vi "FTW-Request-ReplyToPoisonPill.vi"(0 "Poison Pill Request":refnum<data-value>, 5 "Shutting Down?":bool=TRUE, 11 "error in":errorcluster) -> (4 "Poison Pill Response":refnum<data-value>, 15 "error out":errorcluster)   [LabVIEW 2014]
doc: "Sends a response message back to the requesting client. This message is attempts to send unconditionally of incoming error. Take caution to wire a sanitized error into this function, because it will be repeated back onto the client. Said another way, an error generated while processing the request will be not only thrown on the request handler, but also on the client as well."
uses:
  json/core/FTW-JSON-Core-Structure.ctl
panel:
  # "Inputs"
  # "Outputs"
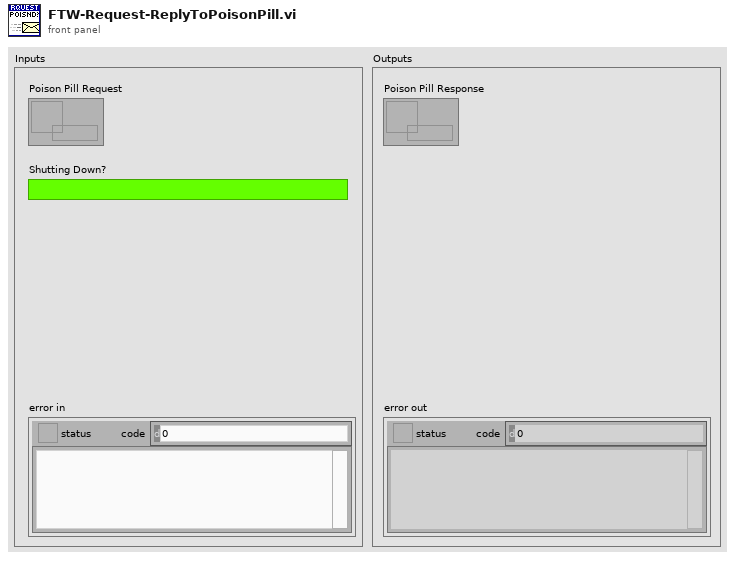
[diagram p1: front panel]
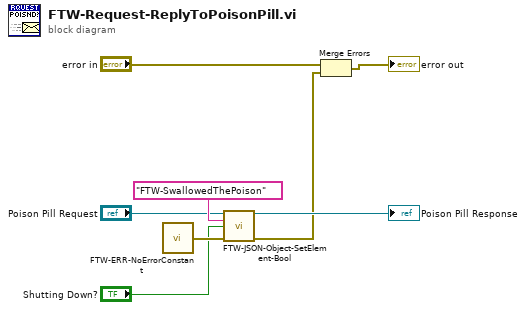
[diagram p0: block diagram]
diagram:
  n1 = call "FTW-ERR-NoErrorConstant.vi"() -> ("no error"=w2:errorcluster)
  n2 = call "FTW-JSON-Object-SetElement-Bool.vi"("JSON Object"="Poison Pill Request", "Key"="FTW-SwallowedThePoison", "Value"="Shutting Down?", "error in"=w2) -> ("JSON Object out"=→"Poison Pill Response":refnum<data-value>, "error out"=w4:errorcluster)  [unwired: 10 in]
  n3 = Merge Errors("error in", w4) -> (→"error out":errorcluster)
